vi "HXG2_CoilData.vi"(8 "error in (no error)":errorcluster, 10 "Fin Data":T2 {"Ext collar length" format="%#.3f in"; "Tubes per plate" format="%#.3f"; "Wire Diameter" format="%#.3f in"; "Fin stretch ratio" format="%#.3f %"; "Fin thickness" format="%#.3f in"; "Fin Width" format="%#.3f in"; "Fin OD" format="%#.3f in"; "Fin contact resistance" format="%#.3f ft² hr °F/BTU"; "Fins per inch (FPI)" format="%#.3f"}, 11 "General_Tube data":T1 {"Tube vertical spacing (Sf)" format="%#.3f in"; "Tube horizontal spacing (Sr)" format="%#.3f in"; "Tube ID" format="%#.3f in"; "Tube thickness" format="%#.3f in"; "Tube OD" format="%#.3f in"; "Tube test Length (tL)" format="%#.3f in"}) -> (0 "error out":errorcluster, 3 "String Data":string[](array[string]))   [LabVIEW 2012]
uses:
  Controls/UI/HXG2_FinData.ctl
  Controls/UI/HXG2_GralTubeData.ctl
panel:
  # "Coil Physical Data"
  # "Spine Fin"
  # "Wire Fin"
  # "Plate Fin"
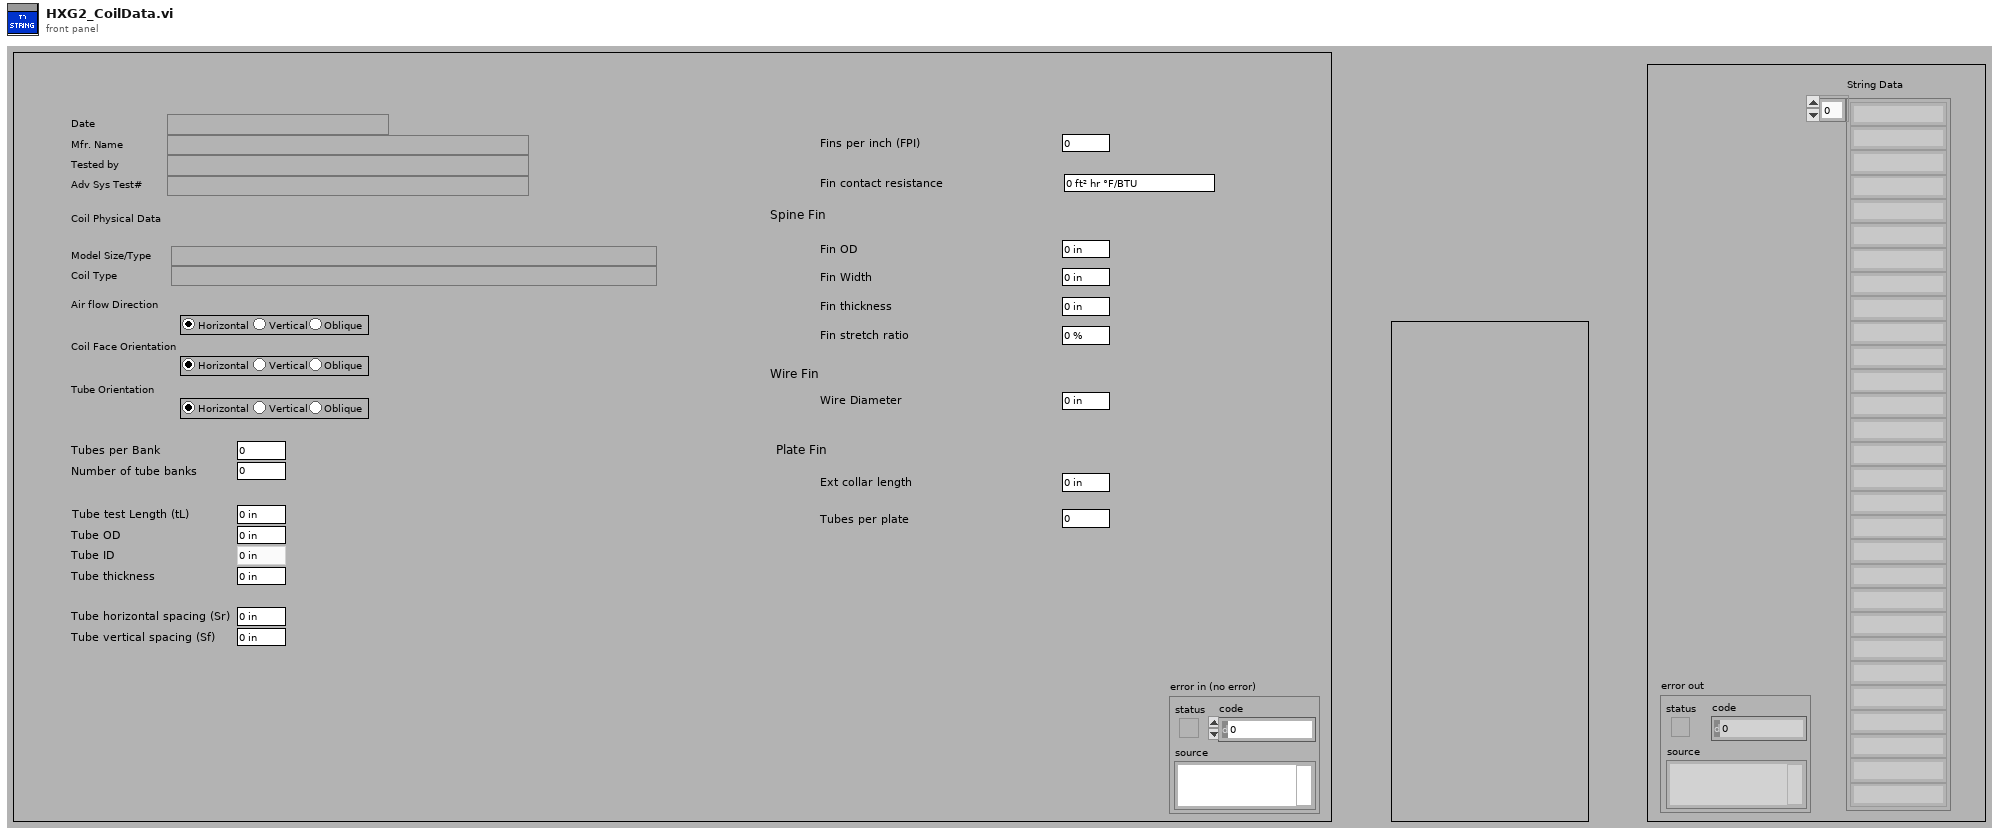
[diagram p1: front panel]
types:
  T1 = typedef "HXG2_GralTubeData.ctl" = cluster{"Date":string, "Mfr. Name":string, "Tested by":string, "Adv Sys Test#":string, "Model Size/Type":string, "Coil Type":string, "Air flow Direction":enum32{"Radio Selection 1", "Radio Selection 2", "Radio Selection 3"}, "Coil Face Orientation":enum32{"Radio Selection 1", "Radio Selection 2", "Radio Selection 3"}, "Tube Orientation":enum32{"Radio Selection 1", "Radio Selection 2", "Radio Selection 3"}, "Tubes per Bank":dbl, "Number of tube banks":dbl, "Tube test Length (tL)":dbl, "Tube OD":dbl, "Tube thickness":dbl, "Tube ID":dbl, "Tube horizontal spacing (Sr)":dbl, "Tube vertical spacing (Sf)":dbl}
  T2 = typedef "HXG2_FinData.ctl" = cluster{"Fins per inch (FPI)":dbl, "Fin contact resistance":dbl, "Fin OD":dbl, "Fin Width":dbl, "Fin thickness":dbl, "Fin stretch ratio":dbl, "Wire Diameter":dbl, "Tubes per plate":dbl, "Ext collar length":dbl}
  T3 = enum32{"Radio Selection 1", "Radio Selection 2", "Radio Selection 3"}
  T4 = enum32{"Radio Selection 1", "Radio Selection 2", "Radio Selection 3"}[]
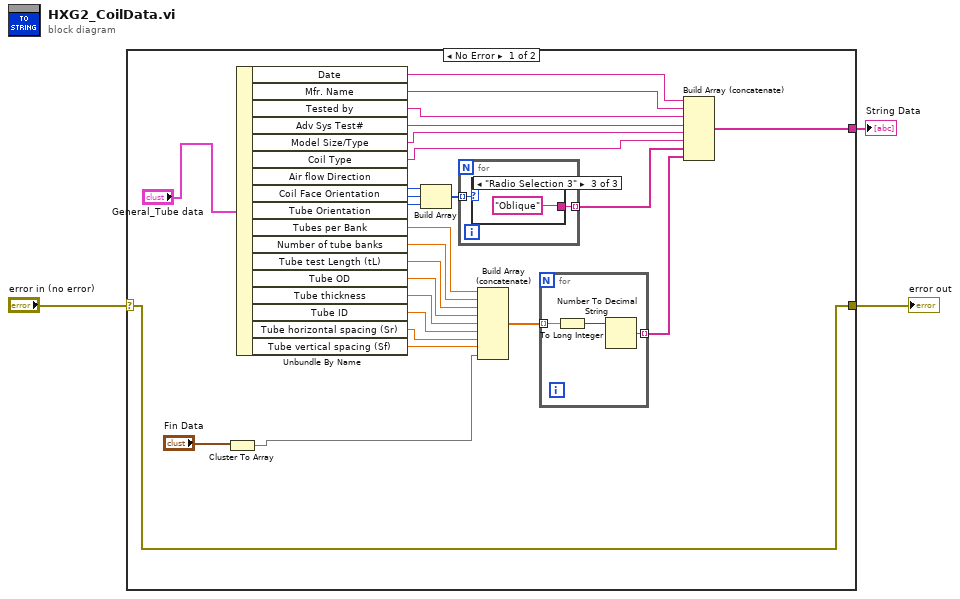
[diagram p0: block diagram]
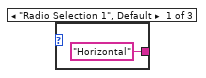
[diagram p2: hidden frame]
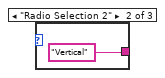
[diagram p3: hidden frame]
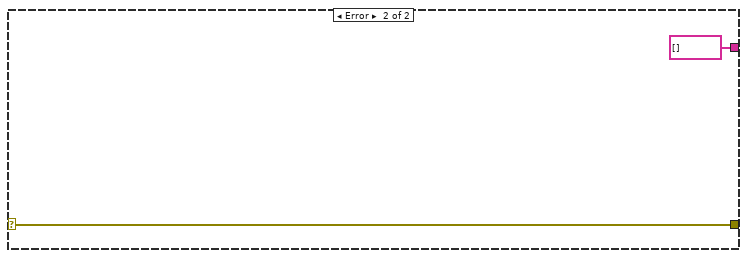
[diagram p4: hidden frame]
diagram:
  n1 = case shown="No Error" "error in (no error)" {
    selector: "error in (no error)" -> [w25 w39]
    tunnel: [w25 w39] -> w3
    tunnel: [w4 string[] []] -> w1
    frame No Error {
      n2 = Cluster To Array(cluster="Fin Data") -> (array=w7:dbl[])
      n3 = Unbundle By Name("General_Tube data") -> ("Date"=w23:string, "Mfr. Name"=w22:string, "Tested by"=w21:string, "Adv Sys Test#"=w20:string, "Model Size/Type"=w19:string, "Coil Type"=w18:string, "Air flow Direction"=w27:T3, "Coil Face Orientation"=w28:T3, "Tube Orientation"=w29:T3, "Tubes per Bank"=w15:dbl, "Number of tube banks"=w14:dbl, "Tube test Length (tL)"=w13:dbl, "Tube OD"=w12:dbl, "Tube thickness"=w11:dbl, "Tube ID"=w10:dbl, "Tube horizontal spacing (Sr)"=w9:dbl, "Tube vertical spacing (Sf)"=w8:dbl)
      n4 = Build Array(w27, w28, w29) -> (w26:T4)
      n5 = for {
        tunnel: w26 -> [w33] mode=indexing
        tunnel: [w34] -> w17 mode=indexing
        n6 = case shown="\"Radio Selection 3\"" w33 {
          tunnel: ["Horizontal" "Vertical" "Oblique"] -> w34
          frame "Radio Selection 1", Default {
          }
          frame "Radio Selection 2" {
          }
          frame "Radio Selection 3" {
          }
        }
      }
      n7 = Build Array (concatenate)(w15, w14, w13, w12, w11, w10, w9, w8, w7) -> (w6:dbl[])
      n8 = for {
        tunnel: w6 -> [w32] mode=indexing
        tunnel: [w30] -> w5 mode=indexing
        n9 = To Long Integer(number=w32) -> (32bit integer=w31:i32)
        n10 = Number To Decimal String(number=w31) -> (decimal integer string=w30:string)  [unwired: 1 in]
      }
      n11 = Build Array (concatenate)(w23, w22, w21, w20, w19, w18, w17, w5) -> (w4:string[])
    }
    frame Error {
    }
  }
  "error out" <- w3
  "String Data" <- w1
